vi "Release Sequence.vi"(0 "PWM 5 Input":dbl, 2 "AI 5 Feedback":dbl, 3 "PWM 7 Input":dbl, 5 "AI 7 Feedback":dbl, 6 "Extension P":dbl=0.5, 7 "PWM 8 Input":dbl, 8 "Button 8":bool, 9 "PWM 9 Input":dbl, 10 "Enable Release Sequence":bool, 11 "DIO 3":bool) -> (14 "PWM 5 Output":dbl, 16 "PWM 7 Output":dbl, 18 "PWM 8 Output":dbl, 19 "PWM 9 Output":dbl)   [LabVIEW 2011]
uses:
  Robot Global Data.vi
panel:
  in  "PWM 5 Input 2":dbl
  in  "PWM 7 Input 2":dbl
  out "PWM 5 Output 2":dbl
  out "PWM 7 Output 2":dbl
  in  "PWM 8 Input 2":dbl
  out "PWM 8 Output 2":dbl
  in  "Release State 2":dbl
  in  "Enable Release Sequence 2":bool
  in  "AI 5 Feedback 2":dbl
  in  "AI 7 Feedback 2":dbl
  in  "DIO 4":bool
  out "Outer Release State 2":dbl
  in  "PWM 9 Input 2":dbl
  out "PWM 9 Output 2":dbl
  in  "Release Extension Power":dbl=0.2
  in  "Spit Out Speed":dbl=-0.4
  out "AI 5 Current":dbl
  out "AI 7 Current":dbl
  out "Outer Release State":dbl
  in  "Extension Release Extra":dbl=8.0
  in  "Release State":dbl
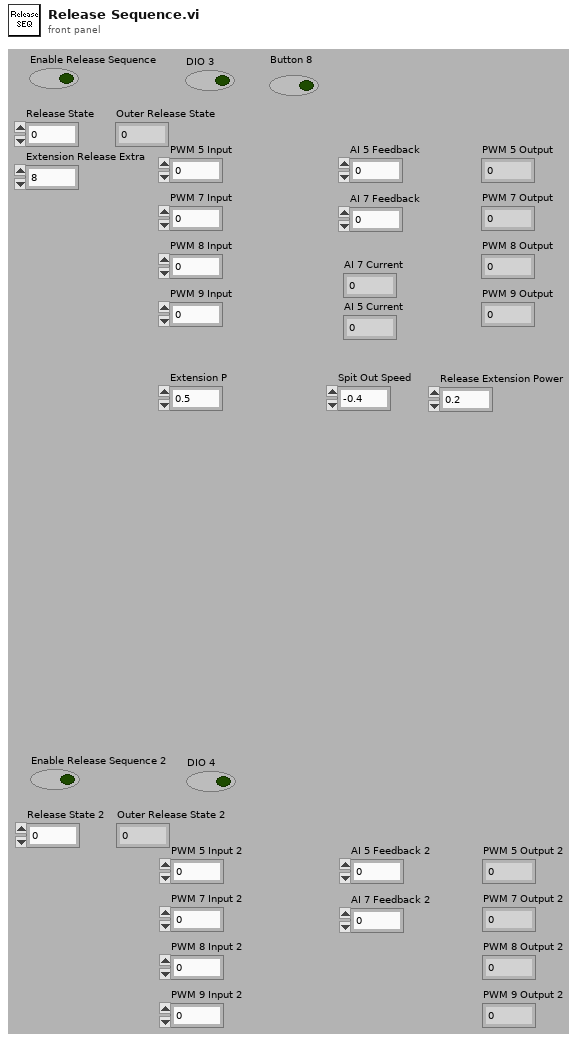
[diagram p1: front panel]
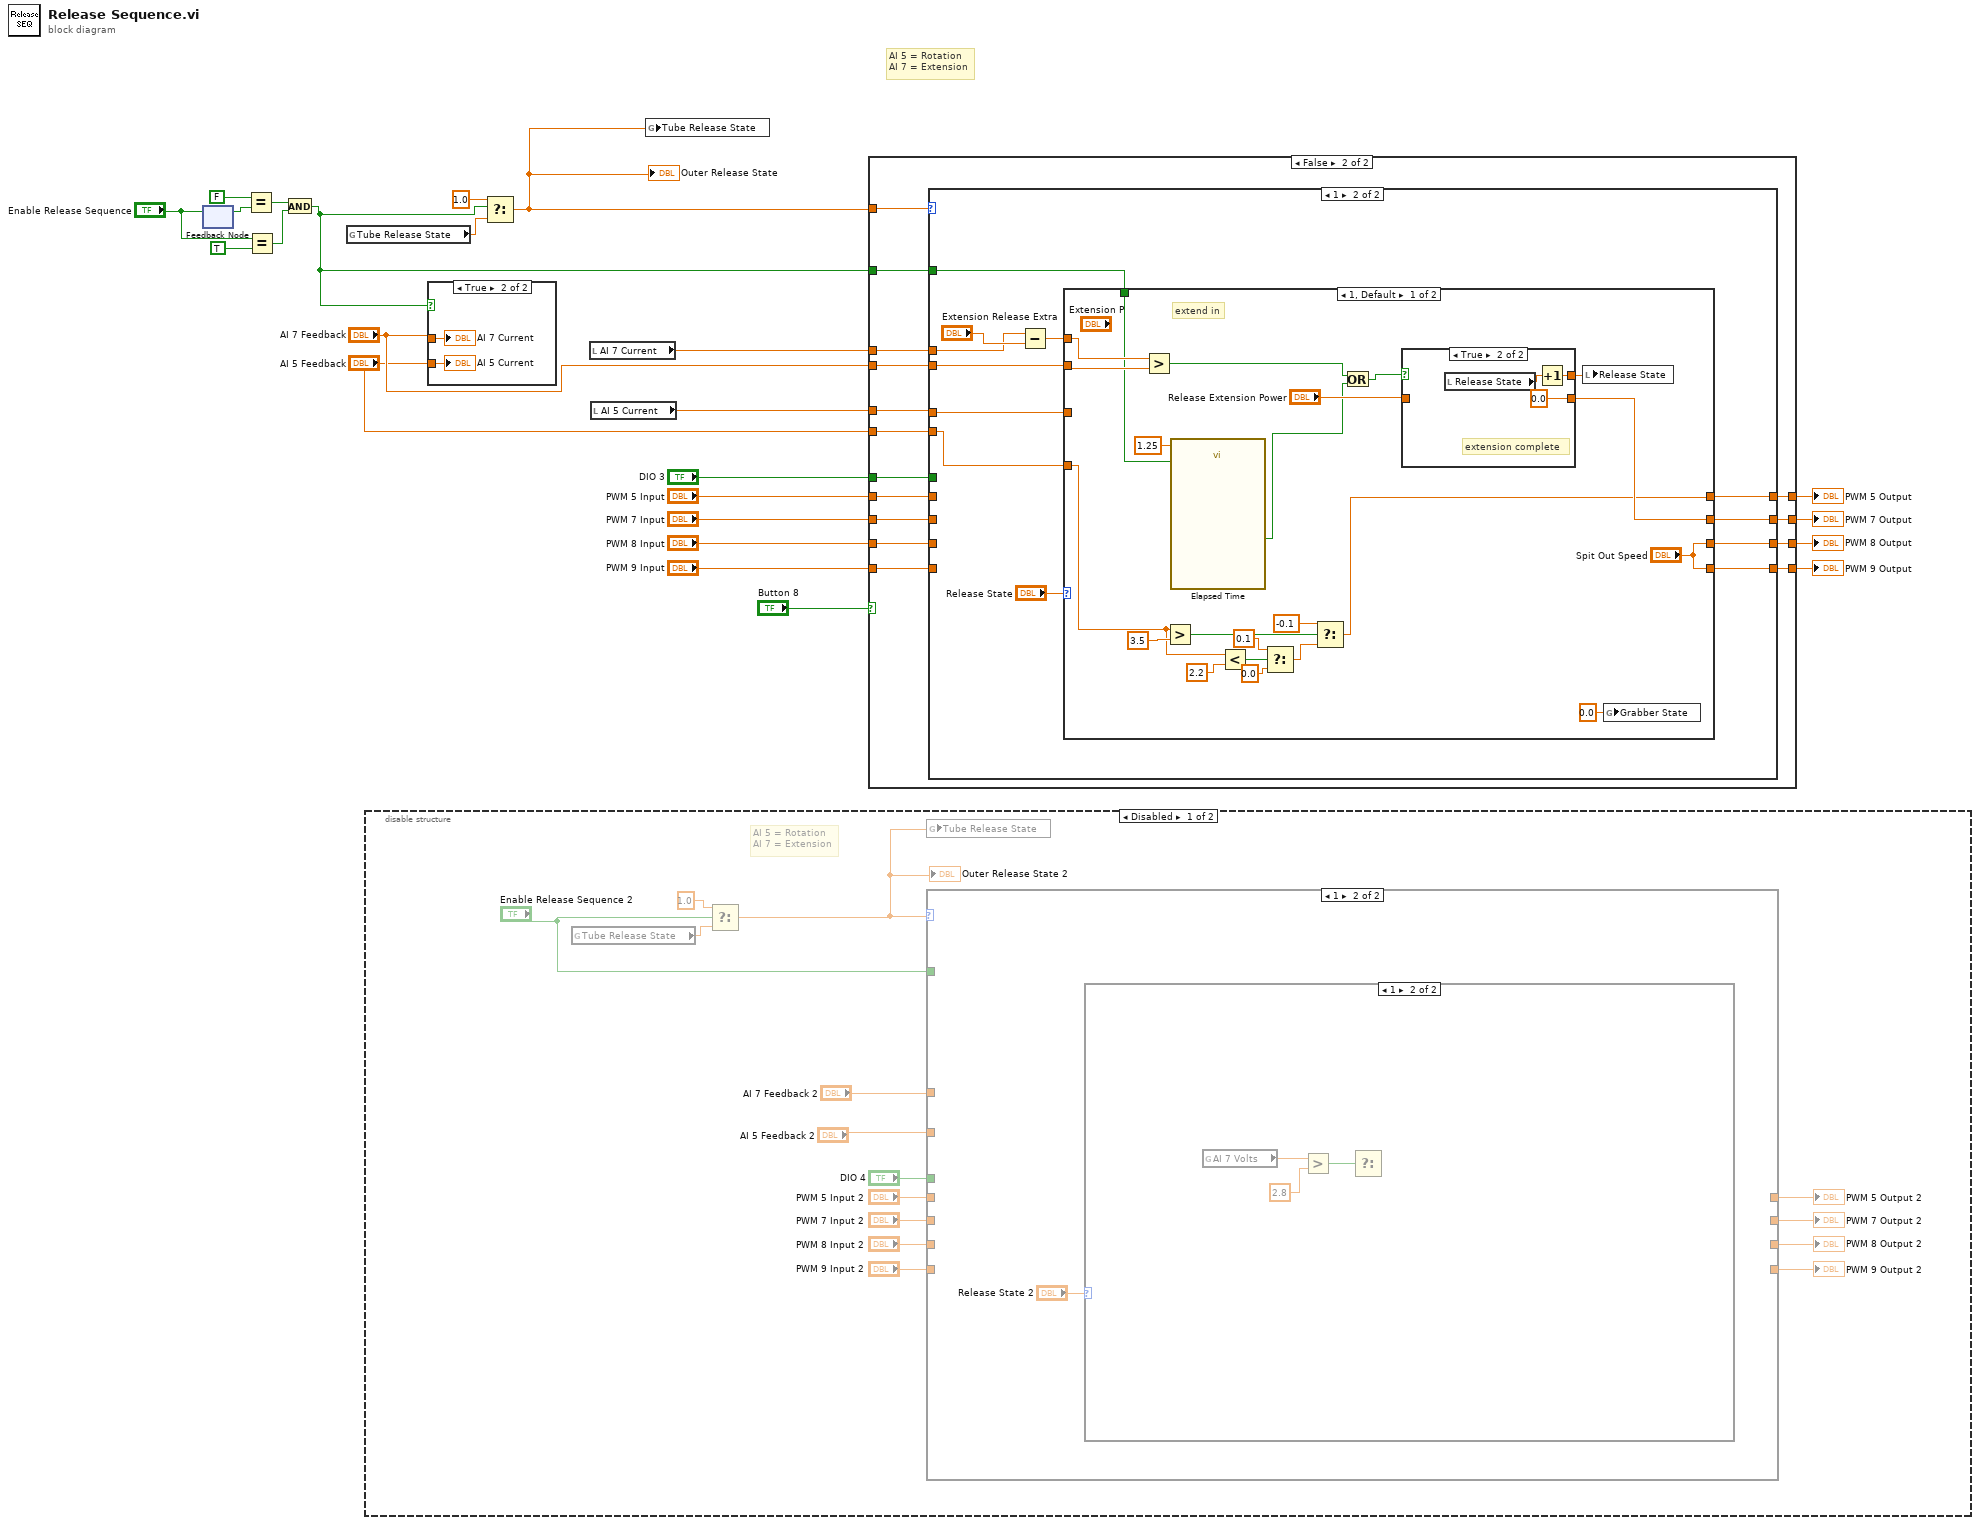
[diagram p0: block diagram]
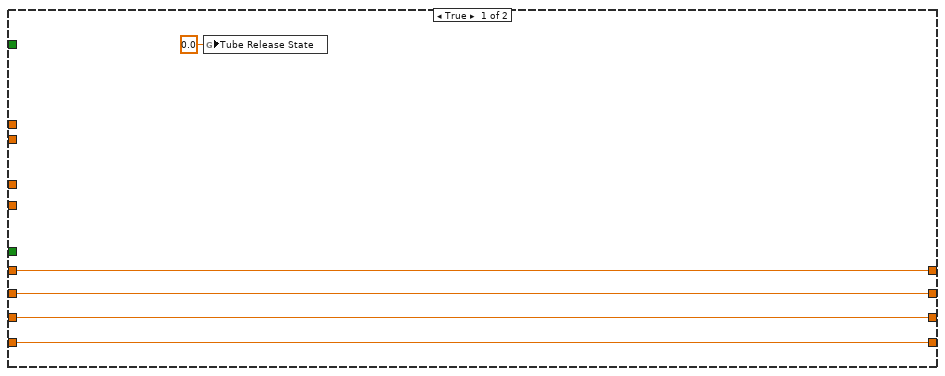
[diagram p2: hidden frame]
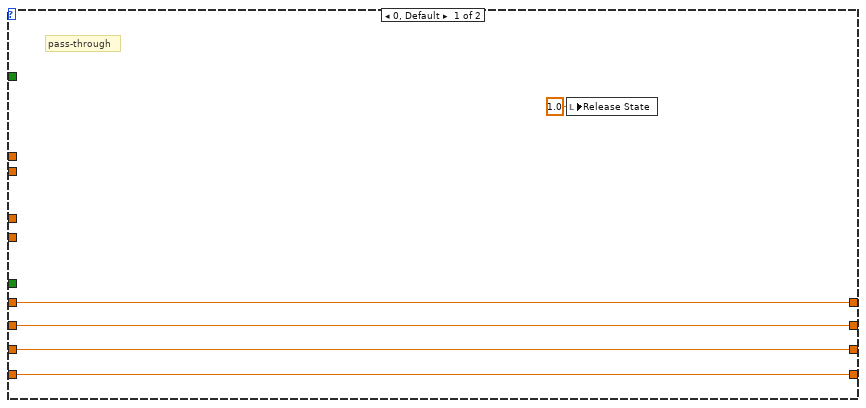
[diagram p3: hidden frame]
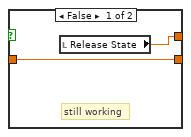
[diagram p4: hidden frame]
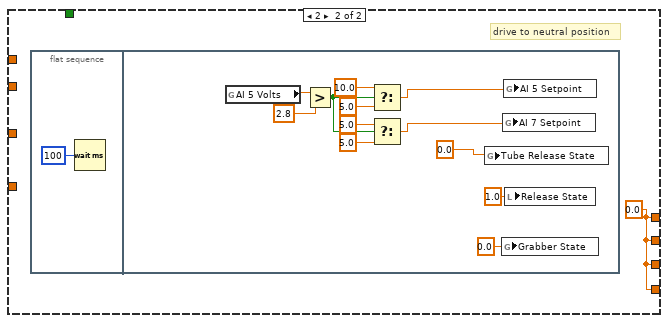
[diagram p5: hidden frame]
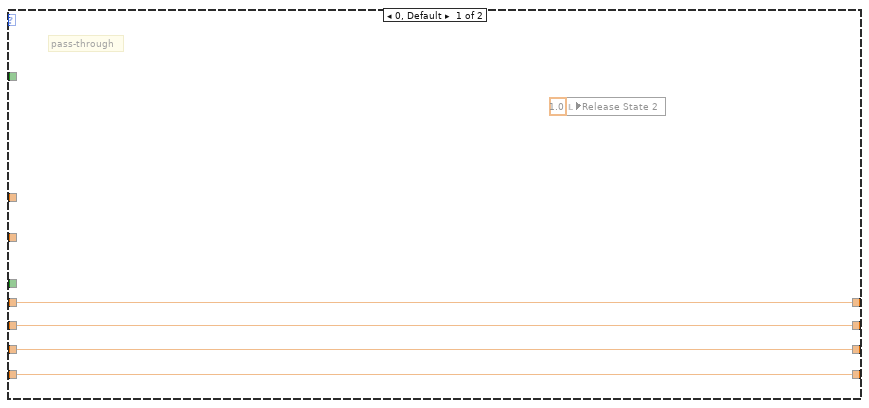
[diagram p7: hidden frame]
diagram:
  # "AI 5 = Rotation\nAI 7 = Extension"
  n1 = feedback-in #1("Enable Release Sequence") -> ()
  n2 = feedback #1() -> (w6:bool)  [unwired: 1 out]
  n3 = Equal?(x=FALSE, y=w6) -> (x = y?=w7:bool)
  n4 = Equal?(x="Enable Release Sequence", y=TRUE) -> (x = y?=w3:bool)
  n5 = And(x=w7, y=w3) -> (x .and. y?=w2:bool)
  n6 = global read "Robot Global Data.vi" "Tube Release State"() -> (w16:dbl)
  n7 = disable-structure shown="Disabled" {
    frame Disabled {
      # "AI 5 = Rotation\nAI 7 = Extension"
      n8 = global read "Robot Global Data.vi" "Tube Release State"() -> (w34:dbl)
      n9 = Select(t=1.0, s="Enable Release Sequence 2", f=w34) -> (s? t:f=w37:dbl)
      "Outer Release State 2" <- w37
      n10 = global write "Robot Global Data.vi" "Tube Release State"(w37) -> ()
      n11 = case shown="1" w37 {
        tunnel: [w44 _] -> w26
        tunnel: "PWM 5 Input 2" -> [w44 _]
        tunnel: "PWM 7 Input 2" -> [w43 _]
        tunnel: [w43 _] -> w29
        tunnel: "PWM 8 Input 2" -> [w42 _]
        tunnel: [w42 _] -> w31
        tunnel: "AI 7 Feedback 2" -> [_ _]
        tunnel: "AI 5 Feedback 2" -> [_ _]
        tunnel: "DIO 4" -> [_ _]
        tunnel: "PWM 9 Input 2" -> [w40 _]
        tunnel: [w40 _] -> w39
        tunnel: "Enable Release Sequence 2" -> [_ _]
        frame 0, Default {
          # "pass-through"
          n12 = local write "Release State 2"(1.0 ("Release State")) -> ()
        }
        frame 1 {
          n13 = case shown="1" "Release State 2" {
            frame 0, Default {
            }
            frame 1 {
              n14 = global read "Robot Global Data.vi" "AI 7 Volts"() -> (w48:dbl)
              n15 = Greater?(x=w48, y=2.8) -> (0:w46:bool)
              n16 = Select(s=w46) -> ()  [unwired: 2 in, 1 out]
            }
          }
        }
      }
      "PWM 5 Output 2" <- w26
      "PWM 7 Output 2" <- w29
      "PWM 8 Output 2" <- w31
      "PWM 9 Output 2" <- w39
    }
    frame Enabled {
    }
  }
  n17 = case shown="True" w2 {
    tunnel: "AI 7 Feedback" -> [_ w50]
    tunnel: "AI 5 Feedback" -> [_ w49]
    frame False {
    }
    frame True {
      "AI 7 Current" <- w50
      "AI 5 Current" <- w49
    }
  }
  n18 = Select(t=1.0, s=w2, f=w16) -> (s? t:f=w11:dbl)
  "Outer Release State" <- w11
  n19 = local read "AI 7 Current"() -> (w12:dbl)
  n20 = local read "AI 5 Current"() -> (w13:dbl)
  n21 = global write "Robot Global Data.vi" "Tube Release State"(w11) -> ()
  n22 = case shown="False" "Button 8" {
    tunnel: [w55 w70] -> w24
    tunnel: "PWM 5 Input" -> [w55 w69]
    tunnel: "PWM 7 Input" -> [w54 w68]
    tunnel: [w54 w67] -> w21
    tunnel: "PWM 8 Input" -> [w53 w66]
    tunnel: [w53 w65] -> w19
    tunnel: "DIO 3" -> [_ w64]
    tunnel: "AI 7 Feedback" -> [_ w63]
    tunnel: "AI 5 Feedback" -> [_ w62]
    tunnel: w13 -> [_ w61]
    tunnel: w12 -> [_ w60]
    tunnel: w11 -> [_ w59]
    tunnel: "PWM 9 Input" -> [w52 w58]
    tunnel: [w52 w57] -> w9
    tunnel: w2 -> [_ w56]
    frame True {
      n23 = global write "Robot Global Data.vi" "Tube Release State"(0.0 ("Tube Release State")) -> ()
    }
    frame False {
      n24 = case shown="1" w59 {
        tunnel: [w75 w82] -> w70
        tunnel: w69 -> [w75 _]
        tunnel: w68 -> [w74 _]
        tunnel: [w74 w84] -> w67
        tunnel: w66 -> [w73 _]
        tunnel: [w73 w80] -> w65
        tunnel: w60 -> [_ w77]
        tunnel: w63 -> [_ w85]
        tunnel: w61 -> [_ w83]
        tunnel: w62 -> [_ w81]
        tunnel: w64 -> [_ _]
        tunnel: w58 -> [w71 _]
        tunnel: [w71 w79] -> w57
        tunnel: w56 -> [_ w76]
        frame 0, Default {
          # "pass-through"
          n25 = local write "Release State"(1.0 ("Release State")) -> ()
        }
        frame 1 {
          n26 = Subtract(x=w77, y="Extension Release Extra") -> (x-y=w86:dbl)
          n27 = case shown="1, Default" "Release State" {
            tunnel: w86 -> [w106 _]
            tunnel: w85 -> [w105 _]
            tunnel: [w109 w115] -> w84
            tunnel: w83 -> [_ _]
            tunnel: [w98 w115] -> w82
            tunnel: w81 -> [w93 _]
            tunnel: ["Spit Out Speed" w115] -> w80
            tunnel: ["Spit Out Speed" w115] -> w79
            tunnel: w76 -> [w89 _]
            frame 1, Default {
              # "extend in"
              n28 = Greater?(x=w106, y=w105) -> (0:w101:bool)
              n29 = Greater?(x=w93, y=3.5) -> (0:w99:bool)
              n30 = call "Elapsed Time"("Time Target (s)"=1.25, "Reset"=w89) -> ("Time has Elapsed"=w96:bool)  [unwired: 3 in, 14 out]
              n31 = Less?(x=w93, y=2.2) -> (x < y?=w94:bool)
              n32 = Select(t=0.1, s=w94, f=0.0) -> (s? t:f=w95:dbl)
              n33 = Select(t=-0.1, s=w99, f=w95) -> (s? t:f=w98:dbl)
              n34 = Or(x=w101, y=w96) -> (x .or. y?=w102:bool)
              n35 = case shown="True" w102 {
                tunnel: [w111 0.0 ("Extension Point 5")] -> w109
                tunnel: "Release Extension Power" -> [w111 _]
                tunnel: [w110 w112] -> w108
                frame False {
                  # "still working"
                  n36 = local read "Release State"() -> (w110:dbl)
                }
                frame True {
                  # "extension complete"
                  n37 = local read "Release State"() -> (w113:dbl)
                  n38 = Increment(x=w113) -> (x+1=w112:dbl)
                }
              }
              n39 = local write "Release State"(w108) -> ()
              n40 = global write "Robot Global Data.vi" "Grabber State"(0.0 ("Grabber State")) -> ()
            }
            frame 2 {
              w115 = 0.0 ("Extension Point 5")
              # "drive to neutral position"
              n41 = flat-sequence {
                frame #0 {
                  n42 = Wait (ms)(milliseconds to wait=u32 100) -> ()  [unwired: 1 out]
                }
                frame #1 {
                  n43 = global read "Robot Global Data.vi" "AI 5 Volts"() -> (w125:dbl)
                  n44 = Greater?(x=w125, y=2.8) -> (0:w119:bool)
                  n45 = Select(t=10.0, s=w119, f=5.0) -> (s? t:f=w120:dbl)
                  n46 = Select(t=5.0, s=w119, f=5.0) -> (s? t:f=w121:dbl)
                  n47 = global write "Robot Global Data.vi" "Tube Release State"(0.0 ("Enable Release Sequence")) -> ()
                  n48 = global write "Robot Global Data.vi" "Grabber State"(0.0 ("Grabber State")) -> ()
                  n49 = global write "Robot Global Data.vi" "AI 7 Setpoint"(w121) -> ()
                  n50 = global write "Robot Global Data.vi" "AI 5 Setpoint"(w120) -> ()
                  n51 = local write "Release State"(1.0 ("Release State")) -> ()
                }
              }
            }
          }
        }
      }
    }
  }
  "PWM 5 Output" <- w24
  "PWM 7 Output" <- w21
  "PWM 8 Output" <- w19
  "PWM 9 Output" <- w9
